vi "REQ full lifecycle v2.vi"(0 "endpoint":string="tcp://127.0.0.1:5555", 1 "Julia ZMQ server file name":string="ZMQ-testserver2.jl", 2 "LV Client state in":T1, 5 "data to send":string="hello", 9 "Force command":bool, 11 "error in":errorcluster, 12 "command":T2, 13 "Jl Server state in":T1) -> (3 "LV Client state out":T1, 6 "server response":string, 14 "Jl Server state out":T1, 15 "error out":errorcluster)   [LabVIEW 2018, in "LV-Julia_ZMQ-Roundtrip_lib.lvlib"]
uses:
  LV-Julia_ZMQ-Roundtrip_lib.lvlib
  Commands v2.ctl
  Server or client state.ctl
  <vilib>/addons/zeromq/zmq_socket.lvclass
  <vilib>/addons/zeromq/zmq_context.lvclass
  commands LV2Jl.ctl
  <vilib>/Utility/error.llb/Error Cluster From Error Code.vi
  <vilib>/ErrorRing/Error Ring.xnode
panel:
  out "return code":i32
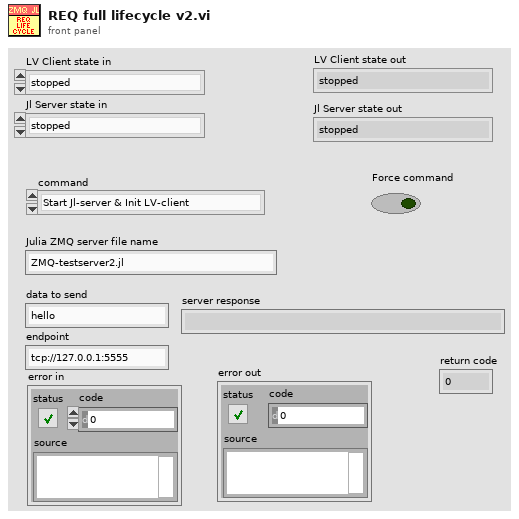
[diagram p1: front panel]
types:
  T1 = typedef "LV-Julia_ZMQ-Roundtrip_lib.lvlib/Server or client state.ctl" = enum16{"stopped", "running", "unknown"}
  T2 = typedef "LV-Julia_ZMQ-Roundtrip_lib.lvlib/Commands v2.ctl" = enum16{"Start Jl-server & Init LV-client", "Send request & Get response ", "Stop Jl-server & Cleanup LV-client", "Cleanup LV-client", "Start Jl-server", "Stop Jl-server", "Init LV-Client", "Cleanup LV-Client", "(not allowed)", "Set LV Client state", "Set Jl Server state"}
  T3 = typedef "commands LV2Jl.ctl" = u8
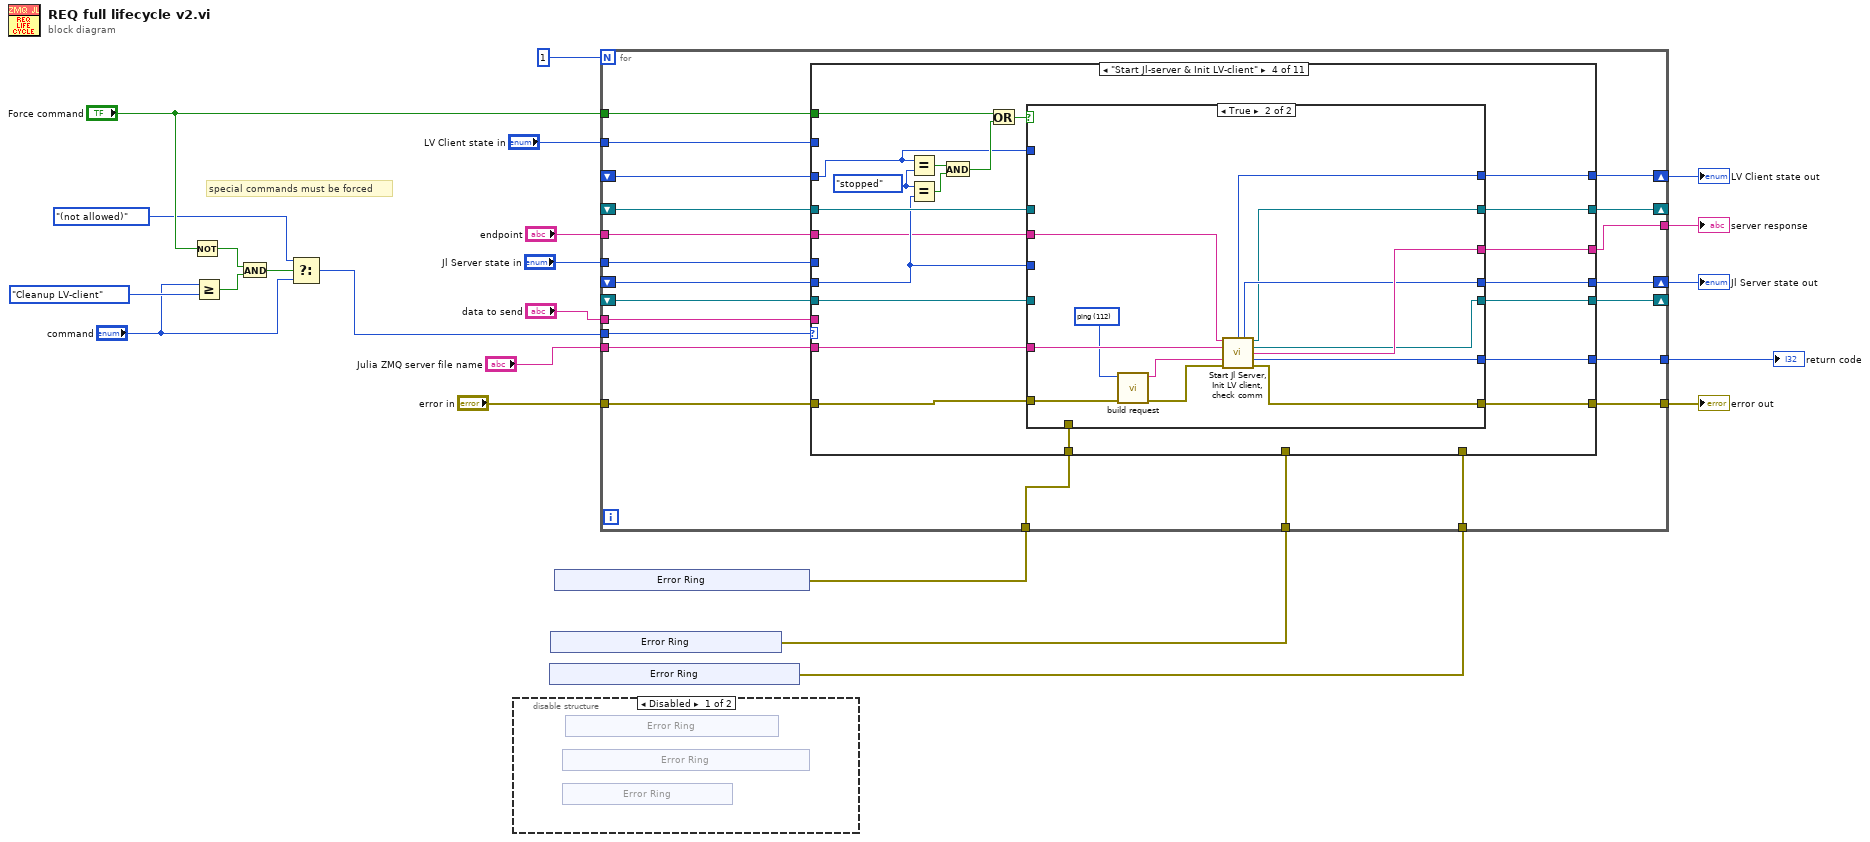
[diagram p0: block diagram]
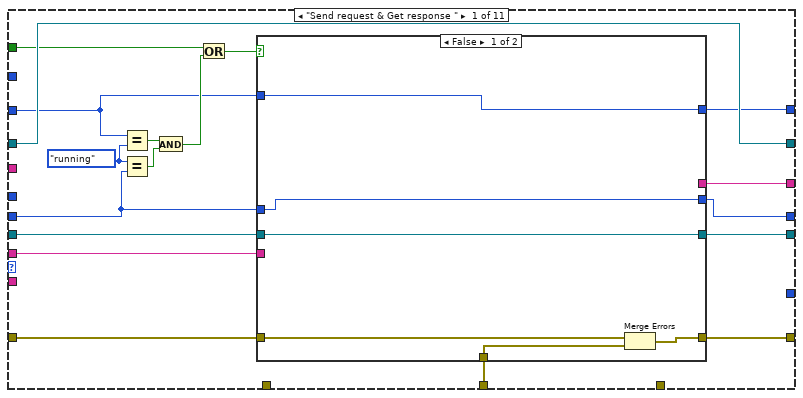
[diagram p3: hidden frame]
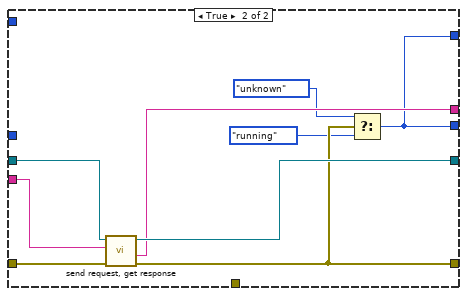
[diagram p4: hidden frame]
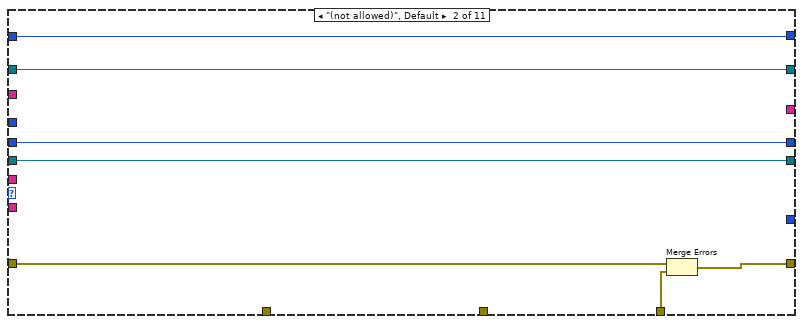
[diagram p5: hidden frame]
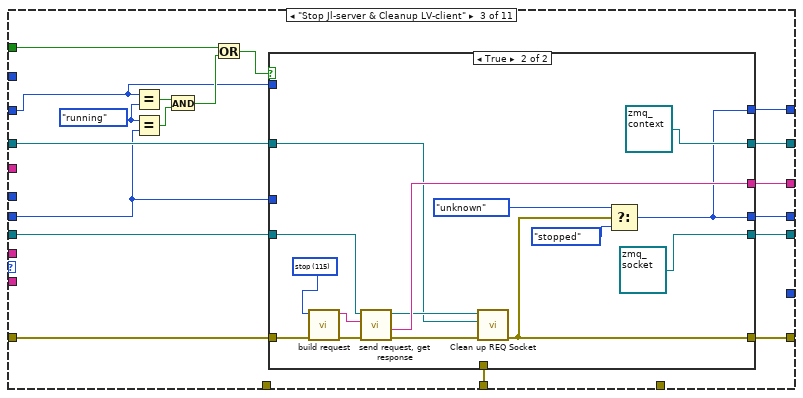
[diagram p6: hidden frame]
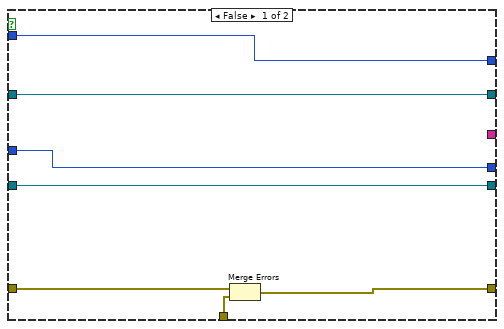
[diagram p7: hidden frame]
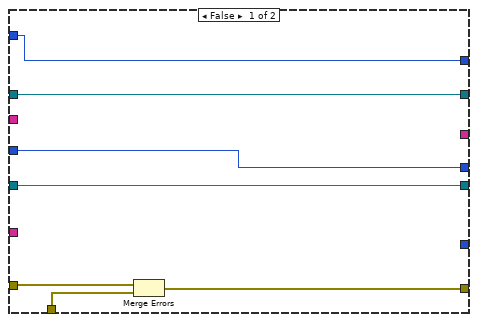
[diagram p8: hidden frame]
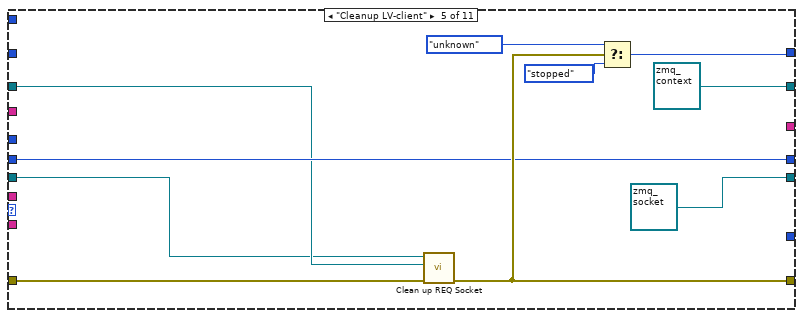
[diagram p9: hidden frame]
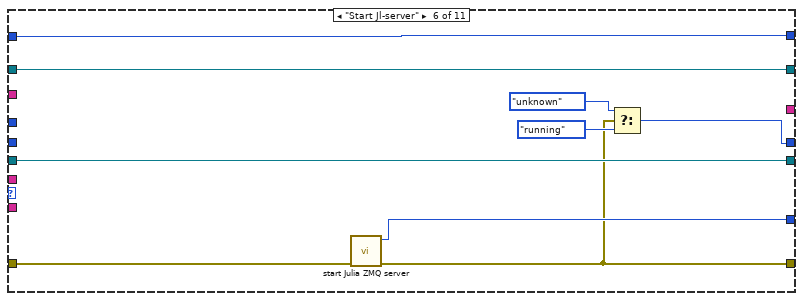
[diagram p10: hidden frame]
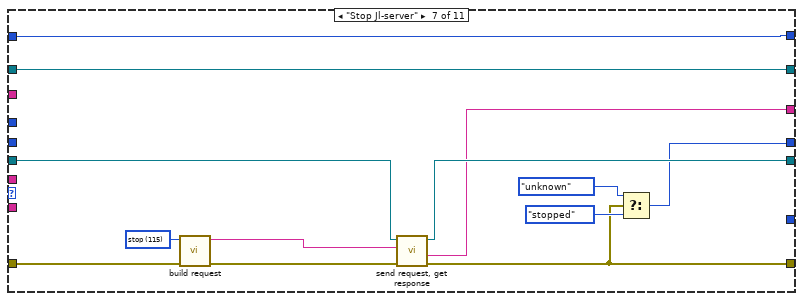
[diagram p11: hidden frame]
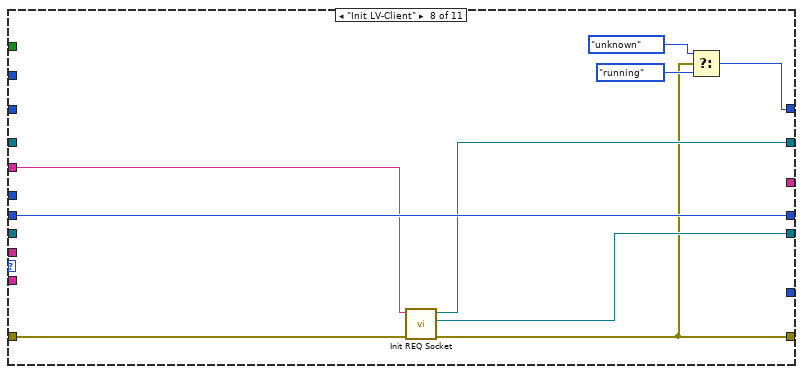
[diagram p12: hidden frame]
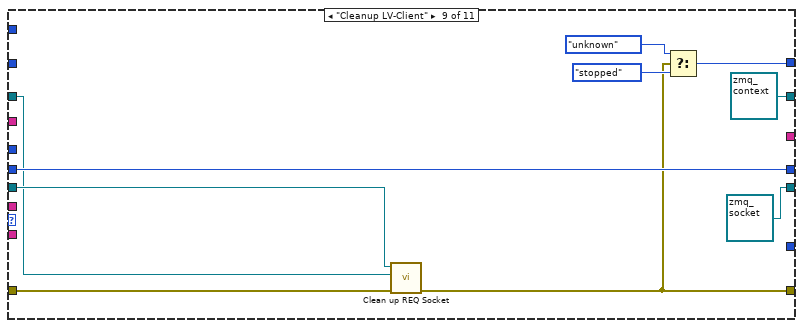
[diagram p13: hidden frame]
diagram:
  # "special commands must be forced"
  n1 = Not(x="Force command") -> (.not. x?=w10:bool)
  n2 = Greater Or Equal?(x="command", y=Commands_v2."Cleanup LV-client" ("command")) -> (x >= y?=w11:bool)
  n3 = And(x=w10, y=w11) -> (x .and. y?=w9:bool)
  n4 = Select(t=Commands_v2."(not allowed)" ("command"), s=w9, f="command") -> (s? t:f=w6:T2)
  n5 = disable-structure shown="Disabled" {
    frame Disabled {
      n6 = xnode "Error Ring"() -> ()  [unwired: 1 out]
      n7 = xnode "Error Ring"() -> ()  [unwired: 1 out]
      n8 = xnode "Error Ring"() -> ()  [unwired: 1 out]
    }
    frame Enabled {
    }
  }
  n9 = xnode "Error Ring"() -> ("error out"=w5:errorcluster)
  n10 = xnode "Error Ring"() -> ("error out"=w14:errorcluster)
  n11 = xnode "Error Ring"() -> ("error out"=w16:errorcluster)
  n12 = for {
    N: 1 -> [_]
    tunnel: [w60] -> w22
    tunnel: [w59] -> w21
    shift-right: [w58] -> _
    shift-left: _ -> [w51]
    tunnel: "endpoint" -> [w57]
    tunnel: "data to send" -> [w56]
    shift-right: [w55] -> _
    shift-left: _ -> [w50]
    tunnel: "error in" -> [w54]
    shift-right: [w52] -> w15
    shift-left: _ -> [w53]
    tunnel: w6 -> [w49]
    tunnel: "Julia ZMQ server file name" -> [w48]
    tunnel: w16 -> [w47]
    tunnel: "Force command" -> [w46]
    shift-right: [w45] -> w4
    shift-left: _ -> [w44]
    tunnel: w14 -> [w43]
    tunnel: w5 -> [w42]
    tunnel: [w41] -> w3
    tunnel: "LV Client state in" -> [w40]
    tunnel: "Jl Server state in" -> [w39]
    n13 = case shown="\"Start Jl-server & Init LV-client\"" w49 {
      tunnel: [w72 w99 w114 w160 w188 w192 w206 w215 w223 w234 w239] -> w60
      tunnel: [w73 _ w116 w149 _ _ w209 _ _ _ _] -> w59
      tunnel: [w78 w96 w111 w157 refnum<class "zmq_context.lvclass"> refnum ("zmq_context out") w197 w211 w217 refnum<class "zmq_context.lvclass"> refnum ("zmq_context out") w237 w241] -> w58
      tunnel: w57 -> [_ _ _ w148 _ _ _ w214 _ _ _]
      tunnel: w56 -> [w74 _ _ _ _ _ _ _ _ _ _]
      tunnel: [w76 w94 w112 w153 refnum<class "zmq_socket.lvclass"> refnum ("zmq_socket out") w196 w210 w216 refnum<class "zmq_socket.lvclass"> refnum ("socket out") w235 w240] -> w55
      tunnel: w54 -> [w77 w100 w118 w161 w191 w199 w203 w218 w226 w234 w239]
      tunnel: [w71 w95 w115 w156 w186 w193 w205 w220 w227 w236 w238] -> w52
      tunnel: w48 -> [_ _ _ w155 _ _ _ _ _ _ _]
      tunnel: w50 -> [w75 w94 w117 w154 w184 w196 w213 _ w225 w235 w240]
      tunnel: w51 -> [w78 w96 w113 w158 w185 w197 w211 _ w224 w237 w241]
      tunnel: w53 -> [w62 w95 w104 w152 w186 _ _ w220 w227 w236 _]
      tunnel: w47 -> [_ _ _ w159 _ _ _ _ _ _ _]
      tunnel: w46 -> [w65 _ w105 w150 _ _ _ _ _ _ _]
      tunnel: [w70 w97 w103 w147 w187 w200 w212 w219 w230 w233 w242] -> w45
      tunnel: w44 -> [w63 w97 w101 w142 _ w200 w212 _ _ _ w242]
      tunnel: w43 -> [w61 _ w102 _ _ _ _ _ _ _ _]
      tunnel: w42 -> [_ w98 _ _ _ _ _ _ _ _ _]
      tunnel: [_ _ _ w141 _ w198 _ _ _ _ _] -> w41
      tunnel: w40 -> [_ _ _ _ _ _ _ _ _ w233 _]
      tunnel: w39 -> [_ _ _ _ _ _ _ _ _ _ w238]
      frame "Send request & Get response " {
        w68 = Server_or_client_state."running" ("Server state")
        n14 = Equal?(x=w63, y=w68) -> (x = y?=w66:bool)
        n15 = Equal?(x=w68, y=w62) -> (x = y?=w69:bool)
        n16 = And(x=w66, y=w69) -> (x .and. y?=w67:bool)
        n17 = Or(x=w65, y=w67) -> (x .or. y?=w64:bool)
        n18 = case shown="False" w64 {
          tunnel: w77 -> [w81 w93]
          tunnel: [w82 w92] -> w76
          tunnel: w75 -> [w82 w91]
          tunnel: w74 -> [_ w90]
          tunnel: [_ w89] -> w73
          tunnel: [w80 w87] -> w72
          tunnel: [w83 w86] -> w71
          tunnel: w62 -> [w83 _]
          tunnel: [w84 w86] -> w70
          tunnel: w63 -> [w84 _]
          tunnel: w61 -> [w79 _]
          frame False {
            n19 = Merge Errors(w81, w79) -> (w80:errorcluster)
          }
          frame True {
            n20 = call "send request, get response.vi"("error in (no error)"=w93, "request"=w90, "zmq_socket in"=w91) -> ("error out"=w87:errorcluster, "response"=w89:string, "zmq_socket out"=w92:refnum<class "zmq_socket.lvclass">)  [unwired: 4 in, 2 out]
            n21 = Select(t=Server_or_client_state."unknown" ("Server state"), s=w87, f=Server_or_client_state."running" ("Server state")) -> (s? t:f=w86:T1)
          }
        }
      }
      frame "(not allowed)", Default {
        n22 = Merge Errors(w100, w98) -> (w99:errorcluster)
      }
      frame "Stop Jl-server & Cleanup LV-client" {
        w109 = Server_or_client_state."running" ("Server state")
        n23 = Equal?(x=w101, y=w109) -> (x = y?=w107:bool)
        n24 = Equal?(x=w109, y=w104) -> (x = y?=w110:bool)
        n25 = And(x=w107, y=w110) -> (x .and. y?=w108:bool)
        n26 = Or(x=w105, y=w108) -> (x .or. y?=w106:bool)
        n27 = case shown="True" w106 {
          tunnel: w118 -> [w121 w128]
          tunnel: w117 -> [w123 w140]
          tunnel: [_ w139] -> w116
          tunnel: [w125 w130] -> w115
          tunnel: [w120 w136] -> w114
          tunnel: w113 -> [w122 w133]
          tunnel: [w123 refnum<class "zmq_socket.lvclass"> refnum ("zmq_socket out")] -> w112
          tunnel: [w122 refnum<class "zmq_context.lvclass"> refnum ("zmq_context out")] -> w111
          tunnel: w104 -> [w125 _]
          tunnel: [w124 w130] -> w103
          tunnel: w101 -> [w124 _]
          tunnel: w102 -> [w119 _]
          frame False {
            n28 = Merge Errors(w121, w119) -> (w120:errorcluster)
          }
          frame True {
            w127 = T3 115 items=["call function"=99, "ping"=112, "stop"=115] ("Command")
            n29 = call "build request.vi"("error in (no error)"=w128, "Command"=w127) -> ("error out"=w129:errorcluster, "REQ string"=w126:string)  [unwired: 8 in]
            n30 = call "send request, get response.vi"("error in (no error)"=w129, "request"=w126, "zmq_socket in"=w140) -> ("error out"=w137:errorcluster, "response"=w139:string, "zmq_socket out"=w134:refnum<class "zmq_socket.lvclass">)  [unwired: 4 in, 2 out]
            n31 = call "Clean up REQ Socket.vi"("error in (no error)"=w137, "zmq_context in"=w133, "zmq_socket in"=w134) -> ("error out"=w136:errorcluster)  [unwired: 8 in]
            n32 = Select(t=Server_or_client_state."unknown" ("Server state"), s=w136, f=Server_or_client_state."stopped") -> (s? t:f=w130:T1)
          }
        }
      }
      frame "Start Jl-server & Init LV-client" {
        w145 = Server_or_client_state."stopped" ("Server state")
        n33 = Equal?(x=w142, y=w145) -> (x = y?=w143:bool)
        n34 = Equal?(x=w145, y=w152) -> (x = y?=w146:bool)
        n35 = And(x=w143, y=w146) -> (x .and. y?=w144:bool)
        n36 = Or(x=w150, y=w144) -> (x .or. y?=w151:bool)
        n37 = case shown="True" w151 {
          tunnel: w161 -> [w168 w171]
          tunnel: [w167 w181] -> w160
          tunnel: w159 -> [w166 _]
          tunnel: [w165 w176] -> w157
          tunnel: w158 -> [w165 _]
          tunnel: [w164 w177] -> w156
          tunnel: w152 -> [w164 _]
          tunnel: w155 -> [_ w180]
          tunnel: [w163 w175] -> w153
          tunnel: w154 -> [w163 _]
          tunnel: [_ w179] -> w149
          tunnel: w148 -> [_ w178]
          tunnel: [w162 w174] -> w147
          tunnel: w142 -> [w162 _]
          tunnel: [_ w173] -> w141
          frame False {
            n38 = Merge Errors(w168, w166) -> (w167:errorcluster)
          }
          frame True {
            w170 = T3 112 items=["call function"=99, "ping"=112, "stop"=115] ("Command")
            n39 = call "build request.vi"("error in (no error)"=w171, "Command"=w170) -> ("error out"=w172:errorcluster, "REQ string"=w169:string)  [unwired: 8 in]
            n40 = call "Start Jl Server, Init LV client, check comm.vi"("endpoint"=w178, "Julia ZMQ server file name"=w180, "request"=w169, "error in (no error)"=w172) -> ("LV client state"=w174:T1, "JL server state"=w177:T1, "zmq_context out"=w176:refnum<class "zmq_context.lvclass">, "zmq_socket out"=w175:refnum<class "zmq_socket.lvclass">, "response"=w179:string, "return code"=w173:i32, "error out"=w181:errorcluster)  [unwired: 5 in]
          }
        }
      }
      frame "Cleanup LV-client" {
        n41 = call "Clean up REQ Socket.vi"("error in (no error)"=w191, "zmq_context in"=w185, "zmq_socket in"=w184) -> ("error out"=w188:errorcluster)  [unwired: 8 in]
        n42 = Select(t=Server_or_client_state."unknown" ("Server state"), s=w188, f=Server_or_client_state."stopped") -> (s? t:f=w187:T1)
      }
      frame "Start Jl-server" {
        n43 = call "start Julia ZMQ server.vi"("error in (no error)"=w199) -> ("error out"=w192:errorcluster, "return code"=w198:i32)  [unwired: 9 in]
        n44 = Select(t=Server_or_client_state."unknown" ("Server state"), s=w192, f=Server_or_client_state."running") -> (s? t:f=w193:T1)
      }
      frame "Stop Jl-server" {
        w202 = T3 115 items=["call function"=99, "ping"=112, "stop"=115] ("Command")
        n45 = call "build request.vi"("error in (no error)"=w203, "Command"=w202) -> ("error out"=w204:errorcluster, "REQ string"=w201:string)  [unwired: 8 in]
        n46 = call "send request, get response.vi"("error in (no error)"=w204, "request"=w201, "zmq_socket in"=w213) -> ("error out"=w206:errorcluster, "response"=w209:string, "zmq_socket out"=w210:refnum<class "zmq_socket.lvclass">)  [unwired: 4 in, 2 out]
        n47 = Select(t=Server_or_client_state."unknown" ("Server state"), s=w206, f=Server_or_client_state."stopped") -> (s? t:f=w205:T1)
      }
      frame "Init LV-Client" {
        n48 = call "Init REQ Socket.vi"("error in (no error)"=w218, "endpoint"=w214) -> ("error out"=w215:errorcluster, "socket out"=w216:refnum<class "zmq_socket.lvclass">, "zmq_context out"=w217:refnum<class "zmq_context.lvclass">)  [unwired: 7 in]
        n49 = Select(t=Server_or_client_state."unknown" ("Server state"), s=w215, f=Server_or_client_state."running") -> (s? t:f=w219:T1)
      }
      frame "Cleanup LV-Client" {
        n50 = call "Clean up REQ Socket.vi"("error in (no error)"=w226, "zmq_context in"=w224, "zmq_socket in"=w225) -> ("error out"=w223:errorcluster)  [unwired: 8 in]
        n51 = Select(t=Server_or_client_state."unknown" ("Server state"), s=w223, f=Server_or_client_state."stopped") -> (s? t:f=w230:T1)
      }
      frame "Set LV Client state" {
      }
      frame "Set Jl Server state" {
      }
    }
  }
  "error out" <- w22
  "server response" <- w21
  "Jl Server state out" <- w15
  "LV Client state out" <- w4
  "return code" <- w3
